vi "S2C_CMD_FormatCmd.vi"(8 "Error In":errorcluster, 9 "TableData":string[](array[string]), 10 "Row":i32, 11 "Data In":string[][](array[string])) -> (0 "Error Out":errorcluster, 3 "Data Out":string[][](array[string]))   [LabVIEW 2015]
doc: "Updates the build table row with the Command, Return, and Parameter values."
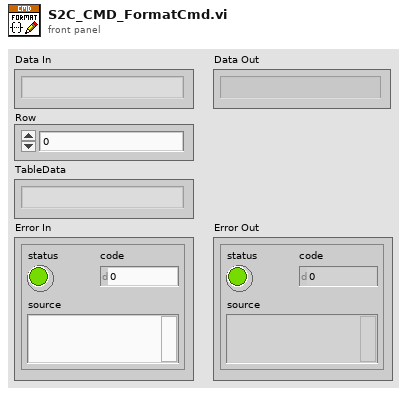
[diagram p1: front panel]
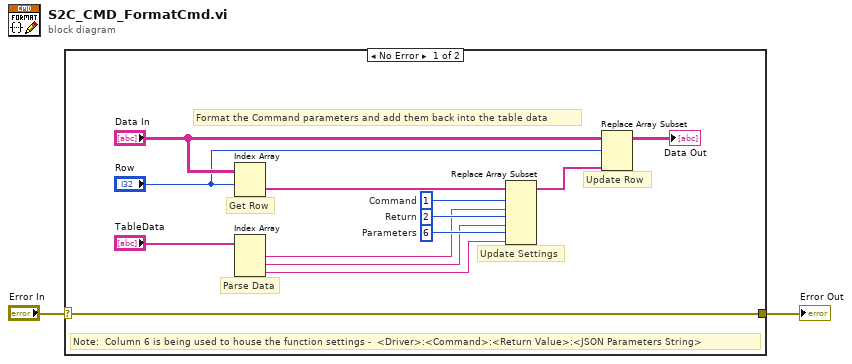
[diagram p0: block diagram]
diagram:
  n1 = case shown="No Error" "Error In" {
    selector: "Error In" -> [w15 w16]
    tunnel: [w15 w16] -> w1
    frame No Error {
      w9 = 6  # Parameters
      w10 = 2  # Return
      w14 = 1  # Command
      # "Parse Data"
      # "Note:  Column 6 is being used to house the function settings -  <Driver>:<Command>:<Return Value>:<JSON Parameters String>"
      # "Update Row"
      # "Update Settings"
      # "Get Row"
      # "Format the Command parameters and add them back into the table data"
      n2 = Index Array(array="Data In", index (row)="Row") -> (element=w5:string[])  [unwired: 1 in]
      n3 = Index Array(array="TableData") -> (element #1=w8:string, element #2=w7:string, element #3=w3:string)  [unwired: 3 in]
      n4 = Replace Array Subset(array=w5, new element #1=w8, index #1=w14, new element #2=w7, index #2=w10, new element #3=w3, index #3=w9) -> (w6:string[])
      n5 = Replace Array Subset(array="Data In", new element=w6, index (row)="Row") -> (→"Data Out":string[][])  [unwired: 1 in]
    }
    frame Error {
    }
  }
  "Error Out" <- w1
